vi "AutoRotatePID.vi"(6 "Timeout (ms)":u32, 8 "error in":errorcluster, 9 "DesiredAngle":dbl format="%#_13g") -> (0 "error out":errorcluster)   [LabVIEW 2013]
doc: "Uses a PID to rotate the robot from the actual angle to the desired angle. The VI returns values for tank drive left and right which can be fed directly into tank drive."
uses:
  Example_Code/Gyro/Read Angle Mode.ctl
  <vilib>/Rock Robotics/WPI/RobotDrive/WPI_RobotDriveGetSetRefNum.vi
  <vilib>/addons/control/pid/pid.llb/PID (DBL).vi
  <vilib>/addons/control/pid/NI_PID_pid.lvlib
panel:
  in  "output high":dbl=1.0 format="%#_13g"
  in  "Stabilize Time (ms)":u32
  in  "Dead Band":dbl format="%#_13g"
  in  "PID gains":T1={"proportional gain (Kc)"=1.0, "integral time (Ti, min)"=0.0, "derivative time (Td, min)"=0.0} {"derivative time (Td, min)" format="%.3f"; "integral time (Ti, min)" format="%.3f"; "proportional gain (Kc)" format="%.3f"}
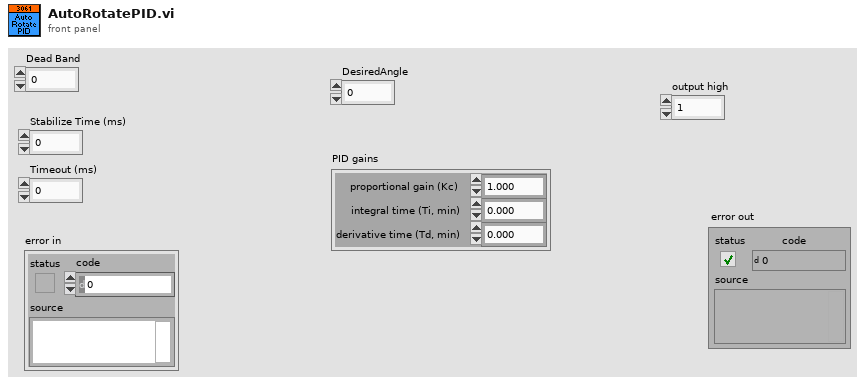
[diagram p1: front panel]
types:
  T1 = cluster{"proportional gain (Kc)":dbl, "integral time (Ti, min)":dbl, "derivative time (Td, min)":dbl}
  T2 = typedef "WPI_RobotDriveDevRef.ctl" = cluster{"DevStatus":errorcluster, "Motors[]":T3[], "Square Inputs":bool, "Max Output":dbl, "Isochronous":bool}
  T3 = typedef "WPI_MotorControlDeviceRef.ctl" = cluster{"DeviceStatus":errorcluster, "Type":enum16{"PWM", "CAN"}, "PWM":cluster{"Digital Module":T4, "PWM Channel":T5, "DeadBand":T6}, "CAN":cluster{"Device Number":u8, "Control Mode":T7, "Semaphore":T8, "Max Vout":dbl}, "Invert":bool, "TransformRef":T9, "InvTransformRef":T9}
  T4 = typedef "FPGA_TypedefDigitalModule.ctl" = enum16{"Digital Module 1", "Digital Module 2"}
  T5 = typedef "FPGA_DIOPWMChannel.ctl" = enum8{"PWM 1", "PWM 2", "PWM 3", "PWM 4", "PWM 5", "PWM 6", "PWM 7", "PWM 8", "PWM 9", "PWM 10", "Invalid"}
  T6 = typedef "WPI_PWMDeadband.ctl" = cluster{"Name":string, "maxPositivePwm":i32, "minPositivePwm":i32, "centerPwm":i32, "maxNegativePwm":i32, "minNegativePwm":i32, "angularRange":u16}
  T7 = typedef "WPI_CANJaguar_ControlMode.ctl" = enum8{"Percent VBus", "Current", "Speed", "Position", "Voltage"}
  T8 = typedef "Semaphore RefNum" = refnum<k1>
  T9 = typedef "WPI_PWMTransform_ConPane.ctl" = refnum<vi>
  T10 = typedef "Read Angle Mode.ctl" = enum16{"Init", "ReadAngle", "Disable"}
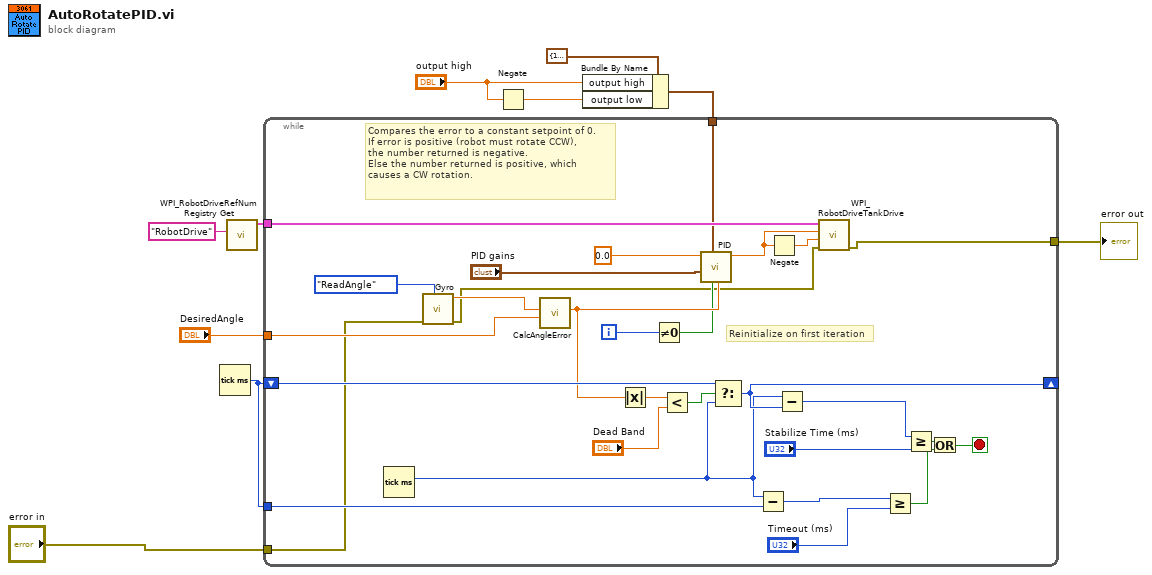
[diagram p0: block diagram]
diagram:
  n1 = Tick Count (ms)() -> (millisecond timer value=w9:u32)
  n2 = call <vilib>:"WPI_RobotDriveRefNum Registry Get.vi"("refnum name"="RobotDrive") -> ("RobotDriveDevRef"=w7:T2)  [unwired: 9 in, 1 out]
  n3 = Negate(x="output high") -> (-x=w6:dbl)
  n4 = Bundle By Name(cluster=cluster{"output high":dbl, "output low":dbl} {"output high"=100.0, "output low"=-100.0} ("output range"), "output high"="output high", "output low"=w6) -> (w3:cluster{"output high":dbl, "output low":dbl})
  n5 = while {
    tunnel: "DesiredAngle" -> [w37]
    shift-right: [w29] -> _
    shift-left: w9 -> [w34]
    tunnel: w9 -> [w24]
    tunnel: w7 -> [w17]
    tunnel: w3 -> [w14]
    tunnel: "error in" -> [w12]
    tunnel: [w11] -> w2
    i -> [w16]
    stop <- w25 stop-if-true
    # "Reinitialize on first iteration"
    # "Compares the error to a constant setpoint of 0.\nIf error is positive (robot must rotate CCW),\nthe number returned is negative.\nElse the number returned is positive, which\ncauses a CW rotation."
    n6 = Tick Count (ms)() -> (millisecond timer value=w23:u32)
    n7 = call "Gyro.vi"("Action"=Read_Angle_Mode."ReadAngle", "error in"=w12) -> ("error out"=w13:errorcluster, "Angle"=w36:dbl)  [unwired: 8 in]
    n8 = call "CalcAngleError.vi"("DesiredAngle"=w37, "ActualAngle"=w36) -> ("Error"=w33:dbl)  [unwired: 9 in]
    n9 = Absolute Value(x=w33) -> (abs(x)=w32:dbl)
    n10 = Not Equal To 0?(x=w16) -> (x != 0?=w15:bool)
    n11 = Less?(x=w32, y="Dead Band") -> (x < y?=w30:bool)
    n12 = call-poly <vilib>:"PID.vi"("reinitialize? (F)"=w15, "output range"=w14, "PID gains"="PID gains", "process variable"=w33, "setpoint"=0.0) -> ("output"=w18:dbl)  [unwired: 5 in, 1 out]
    n13 = Select(t=w34, s=w30, f=w23) -> (s? t:f=w29:u32)
    n14 = Subtract(x=w23, y=w24) -> (x-y=w22:u32)
    n15 = Negate(x=w18) -> (-x=w19:dbl)
    n16 = Subtract(x=w23, y=w29) -> (x-y=w28:u32)
    n17 = call <vilib>:"WPI_RobotDriveTankDrive.vi"("error in (no error)"=w13, "Right axis value"=w19, "Left axis value"=w18, "RobotDriveDevRef"=w17) -> ("error out"=w11:errorcluster)  [unwired: 5 in, 2 out]
    n18 = Greater Or Equal?(x=w22, y="Timeout (ms)") -> (x >= y?=w20:bool)
    n19 = Greater Or Equal?(x=w28, y="Stabilize Time (ms)") -> (x >= y?=w26:bool)
    n20 = Or(x=w26, y=w20) -> (x .or. y?=w25:bool)
  }
  "error out" <- w2
